vi "Gaussian Filter(Pic1 Level1).vi"(1 "Memory In":refnum<k21>, 2 "Data In":u8, 3 "DV In":bool, 6 "Height":u16, 8 "Width":u16, 10 "Rows":u16, 12 "Cols":u16) -> (16 "DV out":bool, 17 "Data Out":fxp<+,8,8>)   [LabVIEW 2016]
uses:
  <vilib>/rvi/DataTransferAndStorage/Container/Common/niFpgaContainerExecOnDevCompGetState.vi
  <vilib>/rvi/Emulation/niFpgaEmulationIsFPGAContextNoSignature.vi
  <vilib>/rvi/DataTransferAndStorage/Container/Common/niFpgaContainerGetUniqueNameForEmu.vi
  <vilib>/rvi/Emulation/niFpgaProcessEmulError.vi
  <vilib>/rvi/Emulation/niFpgaSctlEmulationGetInTimedLoop.vi
  <vilib>/rvi/errors/nirviReportUnexpectedCaseInternalError (U32).vi
  <vilib>/rvi/Memory/Memory_Emulation/niFpgaMemoryEmulationCacheClearOnFirstRun.vi
  <vilib>/rvi/Memory/Memory_Emulation/nirvimemoryEmulationManagerCache_MakeExclusive.vi
  <vilib>/rvi/Memory/Memory_Emulation/niFpgaMemoryEmulationValidateCache.vi
  <vilib>/rvi/Memory/Memory_Emulation/nirvimemoryEmulationManagerCache_InsertValue.vi
  <vilib>/Utility/error.llb/Clear Errors.vi
  <vilib>/rvi/Memory/Memory_Emulation/nirvimemoryEmulationManagerCache_ReleaseExclusive.vi
  <vilib>/rvi/Memory/Memory_Emulation/nirvimemoryEmulationManagerCache_GetValue.vi
  <vilib>/rvi/Memory/Memory_Emulation/nirvimemoryEmulationManagerCache_SetValue.vi
  <vilib>/rvi/Emulation/niFpgaSctlEmulationResourceMgr.vi
  <vilib>/rvi/DataTransferAndStorage/Container/XNode/niFpgaContainer.xnode
  <vilib>/rvi/Memory/Memory_Emulation/niFpgaMemoryEmulationRefIn.vi
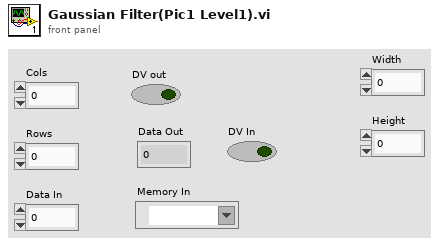
[diagram p1: front panel]
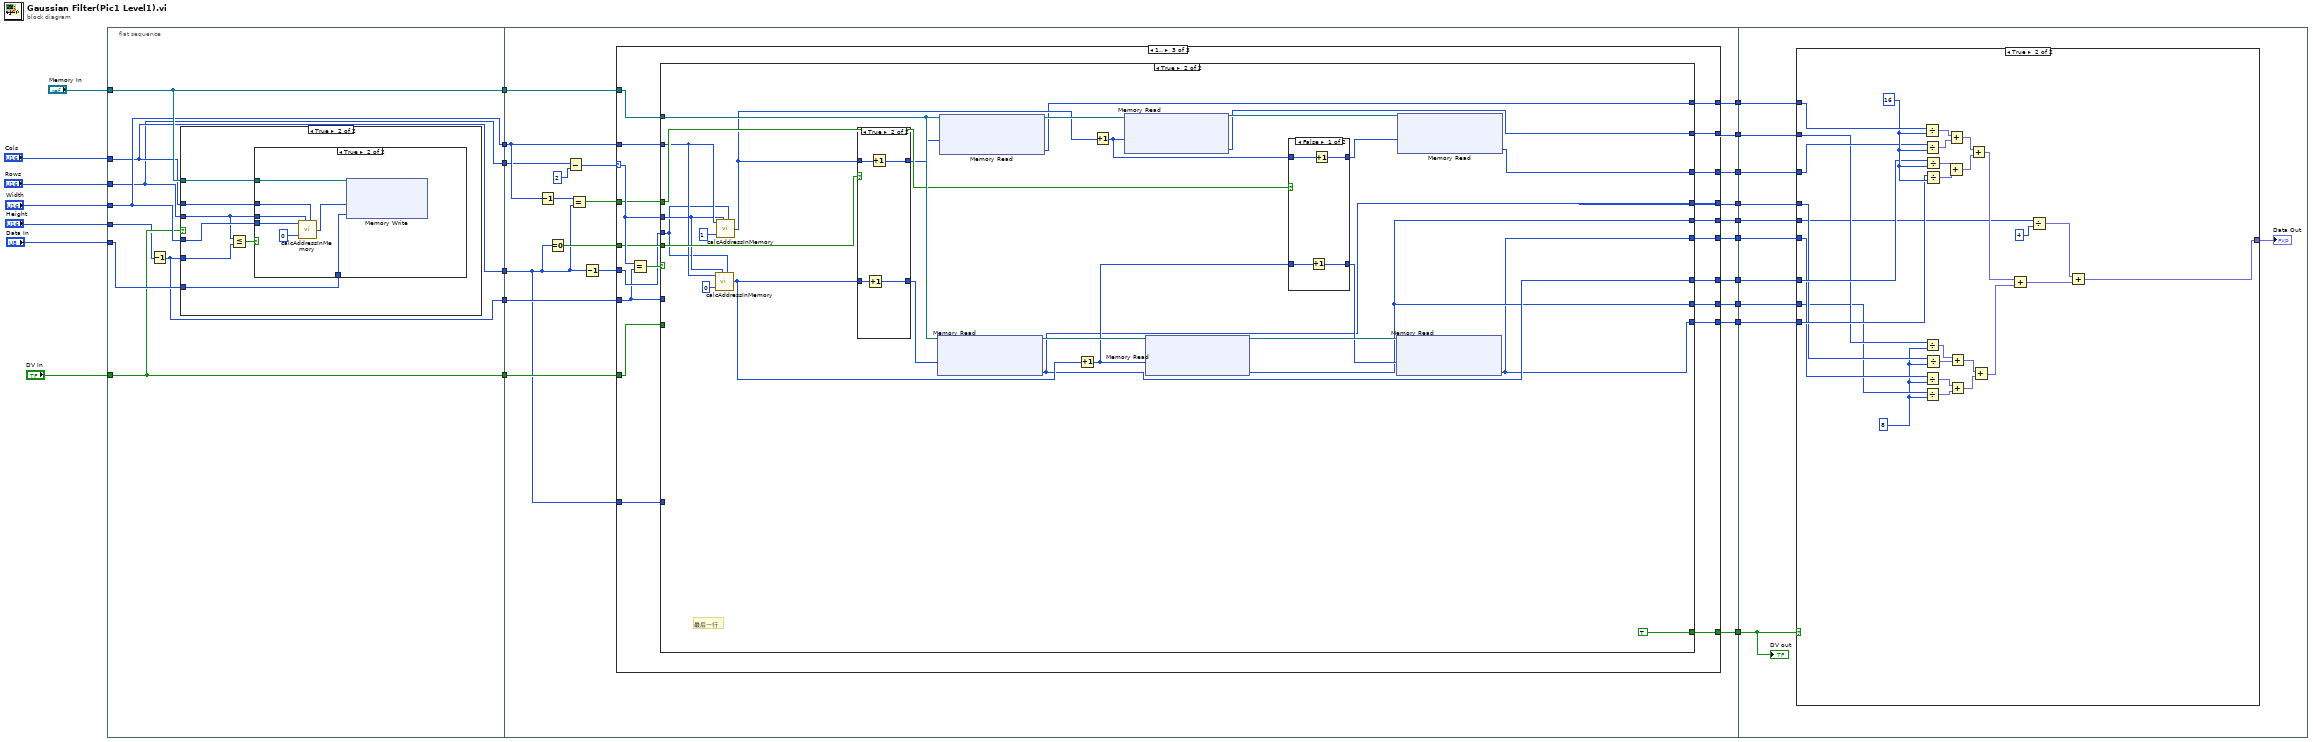
[diagram p0: block diagram]
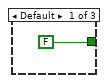
[diagram p4: hidden frame]
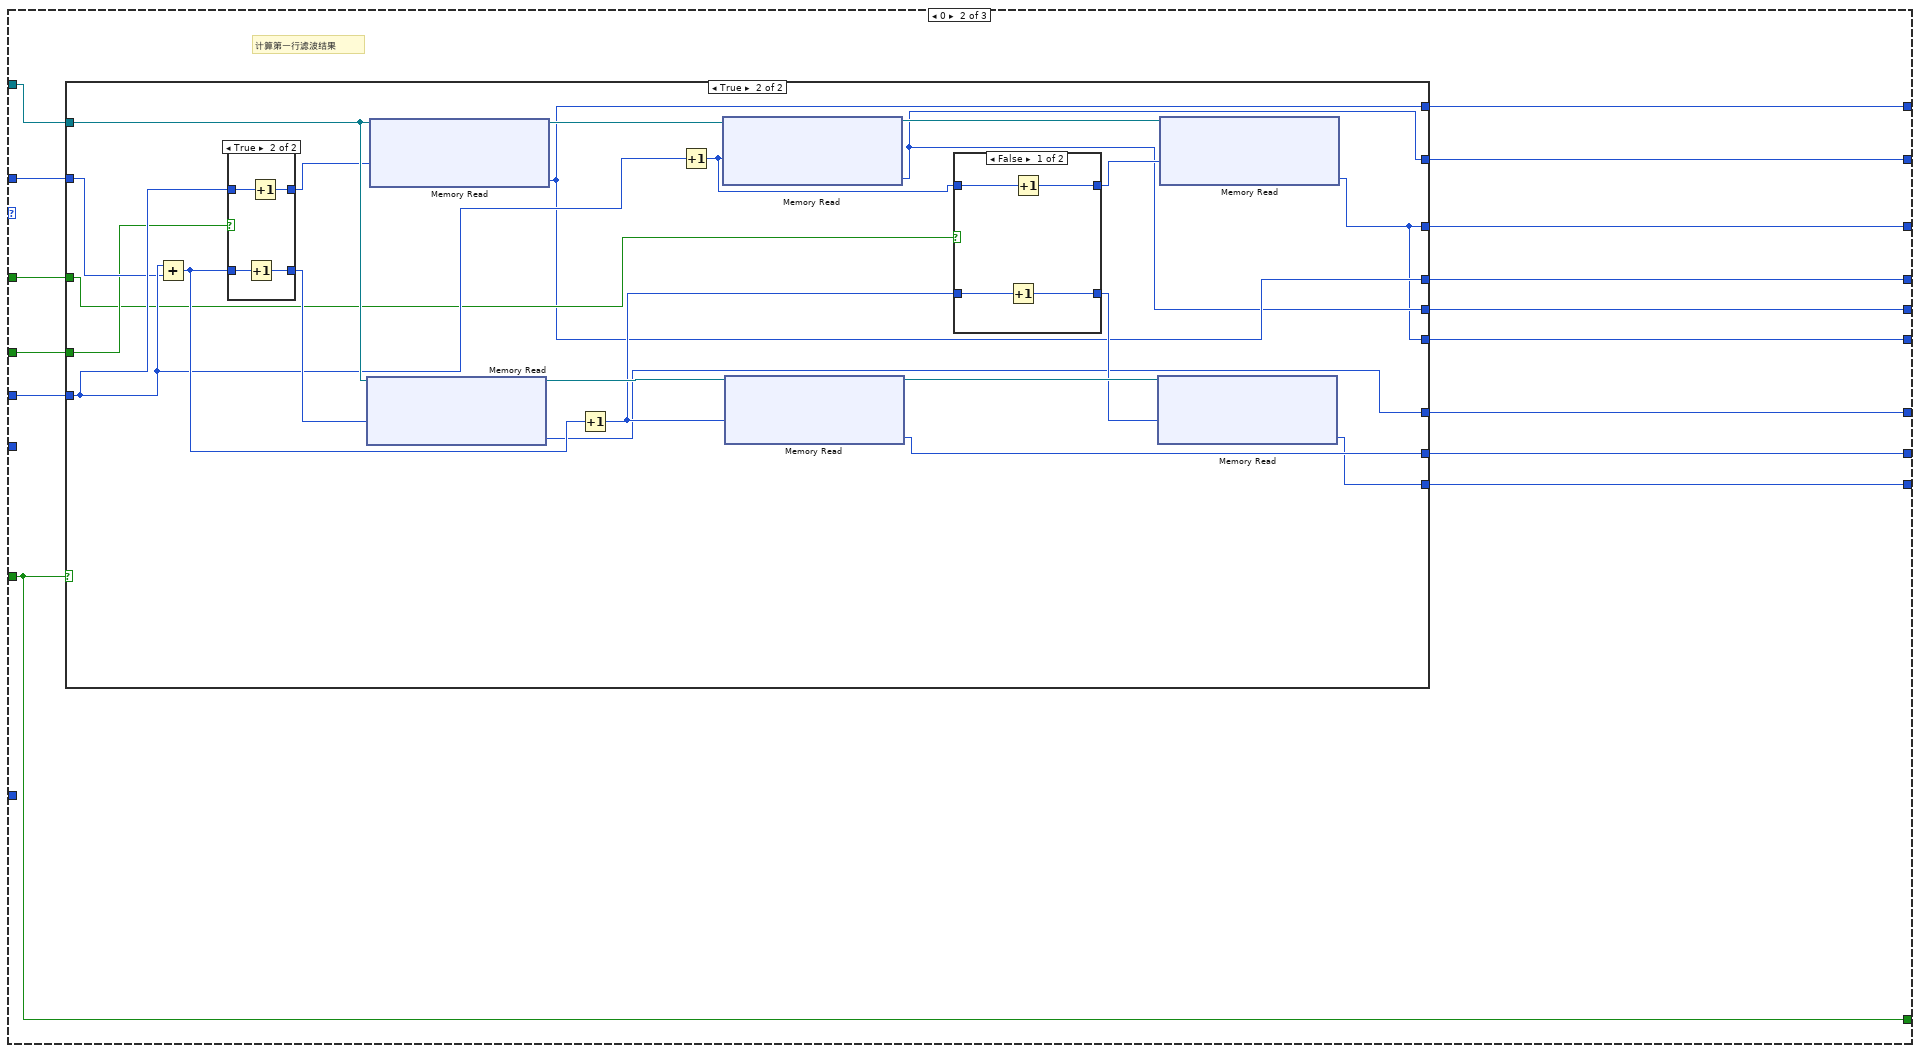
[diagram p5: hidden frame]
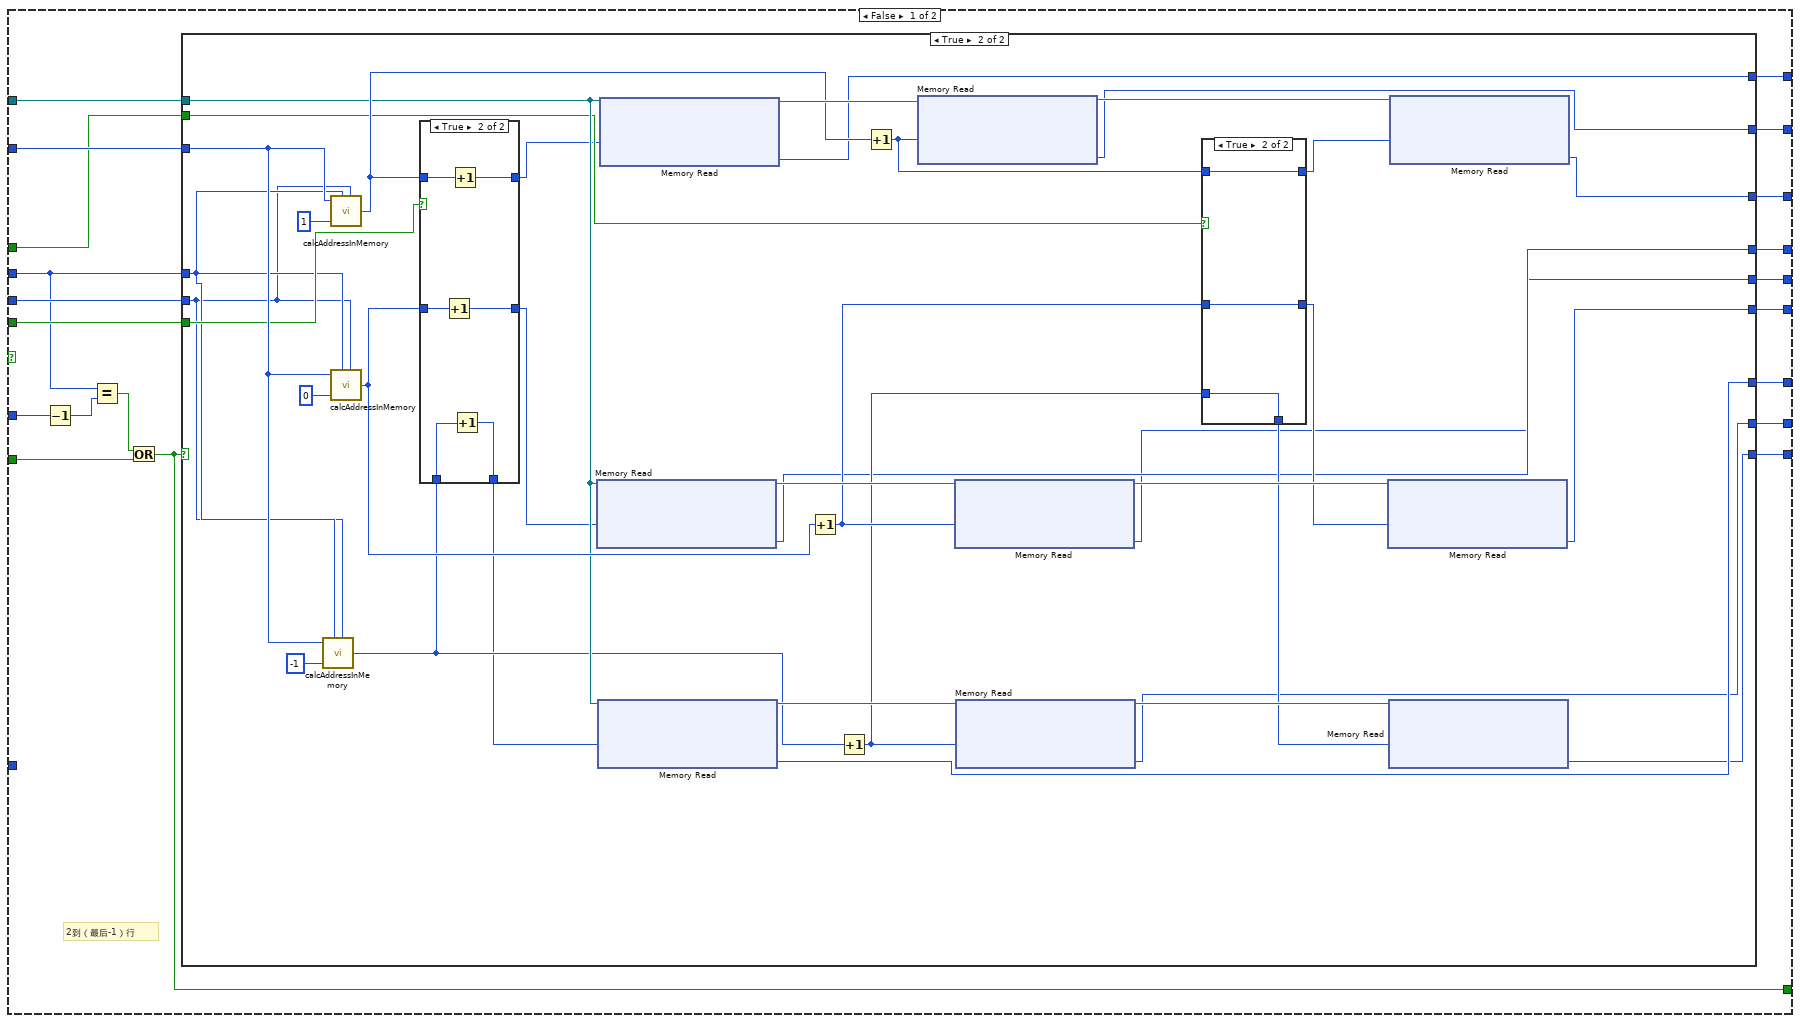
[diagram p9: hidden frame]
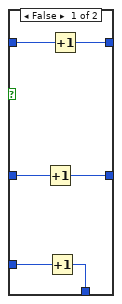
[diagram p11: hidden frame]
diagram:
  n1 = flat-sequence {
    tunnel: [w27] -> w23
    tunnel: [w29] -> w22
    tunnel: [w28] -> w21
    tunnel: [w30] -> w20
    tunnel: [w24] -> w19
    tunnel: [w26] -> w18
    tunnel: "Rows" -> [w27]
    tunnel: "Memory In" -> [w30]
    tunnel: "Cols" -> [w28]
    tunnel: "Data In" -> [w31]
    tunnel: "Width" -> [w29]
    tunnel: "Height" -> [w25]
    tunnel: "DV In" -> [w26]
    tunnel: w23 -> [w49]
    tunnel: w22 -> [w63]
    tunnel: w21 -> [w46]
    tunnel: w20 -> [w67]
    tunnel: w19 -> [w47]
    tunnel: w18 -> [w66]
    tunnel: [w61] -> w10
    tunnel: [w60] -> w9
    tunnel: [w59] -> w8
    tunnel: [w58] -> w7
    tunnel: [w57] -> w6
    tunnel: [w56] -> w5
    tunnel: [w55] -> w4
    tunnel: [w54] -> w3
    tunnel: [w53] -> w2
    tunnel: [w52] -> w1
    tunnel: w10 -> [w260]
    tunnel: w9 -> [w259]
    tunnel: w8 -> [w255]
    tunnel: w7 -> [w258]
    tunnel: w6 -> [w254]
    tunnel: w5 -> [w253]
    tunnel: w4 -> [w252]
    tunnel: w3 -> [w257]
    tunnel: w2 -> [w251]
    tunnel: w1 -> [w256]
    frame #0 {
      n2 = Decrement(x=w25) -> (x-1=w24:u16)
      n3 = case shown="True" w26 {
        tunnel: w31 -> [_ w38]
        tunnel: w27 -> [_ w32]
        tunnel: w29 -> [_ w37]
        tunnel: w28 -> [_ w36]
        tunnel: w30 -> [_ w35]
        tunnel: w24 -> [_ w33]
        frame False {
        }
        frame True {
          n4 = Less Or Equal?(x=w32, y=w33) -> (x <= y?=w34:bool)
          n5 = case shown="True" w34 {
            tunnel: w38 -> [_ w45]
            tunnel: w32 -> [_ w44]
            tunnel: w37 -> [_ w43]
            tunnel: w36 -> [_ w42]
            tunnel: w35 -> [_ w41]
            frame False {
            }
            frame True {
              n6 = call "calcAddressInMemory.vi"("Width"=w43, "Rows"=w44, "delayRowCount"=i16 0, "Cols"=w42) -> ("addressInMemory"=w40:u16)  [unwired: 5 in]
              n7 = xnode ("Memory Write")("Address"=w40, "Data"=w45, "Memory In"=w41) -> ()  [unwired: 1 out]
            }
          }
        }
      }
    }
    frame #1 {
      n8 = Decrement(x=w63) -> (x-1=w62:u16)
      n9 = Equal To 0?(x=w46) -> (x = 0?=w65:bool)
      n10 = Subtract(x=w49, y=i16 2 ("delayRowCount")) -> (x-y=w51:u16)
      n11 = Equal?(x=w62, y=w46) -> (x = y?=w64:bool)
      n12 = Decrement(x=w46) -> (x-1=w50:u16)
      n13 = case shown="1.." w51 {
        selector: w51 -> [_ _ w136]
        tunnel: w67 -> [_ w83 w135]
        tunnel: w50 -> [_ w82 w131]
        tunnel: w63 -> [_ w81 w132]
        tunnel: w47 -> [_ _ w119]
        tunnel: w66 -> [_ w78 w120]
        tunnel: w65 -> [_ w80 w133]
        tunnel: w64 -> [_ w79 w134]
        tunnel: [FALSE w78 w121] -> w61
        tunnel: [_ w77 w130] -> w60
        tunnel: [_ w76 w129] -> w59
        tunnel: [_ w75 w128] -> w58
        tunnel: [_ w74 w127] -> w57
        tunnel: [_ w73 w126] -> w56
        tunnel: [_ w72 w125] -> w55
        tunnel: [_ w71 w124] -> w54
        tunnel: [_ w70 w123] -> w53
        tunnel: [_ w69 w122] -> w52
        tunnel: w46 -> [_ _ w118]
        frame Default {
        }
        frame 0 {
          # "计算第一行滤波结果"
          n14 = case shown="True" w78 {
            tunnel: w83 -> [_ w102]
            tunnel: w82 -> [_ w93]
            tunnel: w81 -> [_ w92]
            tunnel: w80 -> [_ w91]
            tunnel: w79 -> [_ w90]
            tunnel: [_ w89] -> w77
            tunnel: [_ w88] -> w76
            tunnel: [_ w87] -> w75
            tunnel: [_ w89] -> w74
            tunnel: [_ w88] -> w73
            tunnel: [_ w87] -> w72
            tunnel: [_ w86] -> w71
            tunnel: [_ w85] -> w70
            tunnel: [_ w84] -> w69
            frame False {
            }
            frame True {
              n15 = Add(x=w93, y=w92) -> (x+y=w95:u16)
              n16 = case shown="True" w91 {
                tunnel: w93 -> [w113 w117]
                tunnel: [w113 w116] -> w96
                tunnel: w95 -> [w112 w115]
                tunnel: [w112 w114] -> w94
                frame False {
                }
                frame True {
                  n17 = Increment(x=w115) -> (x+1=w114:u16)
                  n18 = Increment(x=w117) -> (x+1=w116:u16)
                }
              }
              n19 = xnode "Memory Read"("Address"=w94, "Memory In"=w102) -> ("Data"=w86:u8, "Memory Out"=w101:refnum<k21>)
              n20 = xnode "Memory Read"("Address"=w96, "Memory In"=w102) -> ("Data"=w89:u8, "Memory Out"=w105:refnum<k21>)
              n21 = Increment(x=w95) -> (x+1=w97:u16)
              n22 = Increment(x=w93) -> (x+1=w98:u16)
              n23 = xnode "Memory Read"("Address"=w98, "Memory In"=w105) -> ("Data"=w88:u8, "Memory Out"=w104:refnum<k21>)
              n24 = xnode "Memory Read"("Address"=w97, "Memory In"=w101) -> ("Data"=w85:u8, "Memory Out"=w100:refnum<k21>)
              n25 = case shown="False" w90 {
                tunnel: [w109 w111] -> w103
                tunnel: [w108 w110] -> w99
                tunnel: w98 -> [w107 w111]
                tunnel: w97 -> [w106 w110]
                frame False {
                  n26 = Increment(x=w106) -> (x+1=w108:u16)
                  n27 = Increment(x=w107) -> (x+1=w109:u16)
                }
                frame True {
                }
              }
              n28 = xnode "Memory Read"("Address"=w99, "Memory In"=w100) -> ("Data"=w84:u8)  [unwired: 1 out]
              n29 = xnode "Memory Read"("Address"=w103, "Memory In"=w104) -> ("Data"=w87:u8)  [unwired: 1 out]
            }
          }
        }
        frame 1.. {
          n30 = Equal?(x=w136, y=w119) -> (x = y?=w137:bool)
          n31 = case shown="True" w137 {
            tunnel: w136 -> [w140 w228]
            tunnel: w135 -> [w157 w234]
            tunnel: w134 -> [w144 w233]
            tunnel: w133 -> [w145 w232]
            tunnel: w132 -> [w155 w229]
            tunnel: w131 -> [w156 w227]
            tunnel: [w154 w217] -> w130
            tunnel: [w153 w216] -> w129
            tunnel: [w152 w215] -> w128
            tunnel: [w151 w214] -> w127
            tunnel: [w150 w213] -> w126
            tunnel: [w149 w212] -> w125
            tunnel: [w148 w214] -> w124
            tunnel: [w147 w213] -> w123
            tunnel: [w146 w212] -> w122
            tunnel: [w143 TRUE] -> w121
            tunnel: w120 -> [w142 _]
            tunnel: w119 -> [w138 _]
            tunnel: w118 -> [_ _]
            frame False {
              # "2到（最后-1）行"
              n32 = Decrement(x=w138) -> (x-1=w139:u16)
              n33 = Equal?(x=w140, y=w139) -> (x = y?=w141:bool)
              n34 = Or(x=w141, y=w142) -> (x .or. y?=w143:bool)
              n35 = case shown="True" w143 {
                tunnel: w157 -> [_ w182]
                tunnel: w156 -> [_ w158]
                tunnel: w155 -> [_ w180]
                tunnel: w140 -> [_ w159]
                tunnel: [_ w168] -> w154
                tunnel: [_ w167] -> w153
                tunnel: [_ w166] -> w152
                tunnel: [_ w165] -> w151
                tunnel: [_ w164] -> w150
                tunnel: [_ w163] -> w149
                tunnel: [_ w162] -> w148
                tunnel: [_ w161] -> w147
                tunnel: [_ w160] -> w146
                tunnel: w145 -> [_ w179]
                tunnel: w144 -> [_ w178]
                frame False {
                }
                frame True {
                  n36 = call "calcAddressInMemory.vi"("Width"=w180, "Rows"=w159, "delayRowCount"=i16 -1, "Cols"=w158) -> ("addressInMemory"=w181:u16)  [unwired: 5 in]
                  n37 = call "calcAddressInMemory.vi"("Width"=w180, "Rows"=w159, "delayRowCount"=i16 1, "Cols"=w158) -> ("addressInMemory"=w186:u16)  [unwired: 5 in]
                  n38 = call "calcAddressInMemory.vi"("Width"=w180, "Rows"=w159, "delayRowCount"=i16 0, "Cols"=w158) -> ("addressInMemory"=w187:u16)  [unwired: 5 in]
                  n39 = case shown="True" w179 {
                    tunnel: w186 -> [w205 w211]
                    tunnel: [w205 w210] -> w177
                    tunnel: w187 -> [w204 w209]
                    tunnel: [w204 w208] -> w174
                    tunnel: [w203 w207] -> w171
                    tunnel: w181 -> [w203 w206]
                    frame False {
                    }
                    frame True {
                      n40 = Increment(x=w209) -> (x+1=w208:u16)
                      n41 = Increment(x=w211) -> (x+1=w210:u16)
                      n42 = Increment(x=w206) -> (x+1=w207:u16)
                    }
                  }
                  n43 = xnode "Memory Read"("Address"=w174, "Memory In"=w182) -> ("Data"=w165:u8, "Memory Out"=w191:refnum<k21>)
                  n44 = xnode "Memory Read"("Address"=w171, "Memory In"=w182) -> ("Data"=w162:u8, "Memory Out"=w184:refnum<k21>)
                  n45 = xnode "Memory Read"("Address"=w177, "Memory In"=w182) -> ("Data"=w168:u8, "Memory Out"=w193:refnum<k21>)
                  n46 = Increment(x=w187) -> (x+1=w173:u16)
                  n47 = Increment(x=w181) -> (x+1=w170:u16)
                  n48 = Increment(x=w186) -> (x+1=w176:u16)
                  n49 = xnode "Memory Read"("Address"=w176, "Memory In"=w193) -> ("Data"=w167:u8, "Memory Out"=w192:refnum<k21>)
                  n50 = xnode "Memory Read"("Address"=w173, "Memory In"=w191) -> ("Data"=w164:u8, "Memory Out"=w190:refnum<k21>)
                  n51 = xnode "Memory Read"("Address"=w170, "Memory In"=w184) -> ("Data"=w161:u8, "Memory Out"=w183:refnum<k21>)
                  n52 = case shown="True" w178 {
                    tunnel: [w199 w202] -> w175
                    tunnel: [w198 w201] -> w172
                    tunnel: w176 -> [w197 w202]
                    tunnel: w173 -> [w196 w201]
                    tunnel: w170 -> [w195 w200]
                    tunnel: [w194 w200] -> w169
                    frame False {
                      n53 = Increment(x=w196) -> (x+1=w198:u16)
                      n54 = Increment(x=w195) -> (x+1=w194:u16)
                      n55 = Increment(x=w197) -> (x+1=w199:u16)
                    }
                    frame True {
                    }
                  }
                  n56 = xnode "Memory Read"("Address"=w172, "Memory In"=w190) -> ("Data"=w163:u8)  [unwired: 1 out]
                  n57 = xnode "Memory Read"("Address"=w169, "Memory In"=w183) -> ("Data"=w160:u8)  [unwired: 1 out]
                  n58 = xnode "Memory Read"("Address"=w175, "Memory In"=w192) -> ("Data"=w166:u8)  [unwired: 1 out]
                }
              }
            }
            frame True {
              # "最后一行"
              n59 = call "calcAddressInMemory.vi"("Width"=w229, "Rows"=w228, "delayRowCount"=i16 0, "Cols"=w227) -> ("addressInMemory"=w226:u16)  [unwired: 5 in]
              n60 = call "calcAddressInMemory.vi"("Width"=w229, "Rows"=w228, "delayRowCount"=i16 1, "Cols"=w227) -> ("addressInMemory"=w225:u16)  [unwired: 5 in]
              n61 = case shown="True" w232 {
                tunnel: w225 -> [w246 w250]
                tunnel: [w246 w249] -> w223
                tunnel: w226 -> [w245 w248]
                tunnel: [w245 w247] -> w220
                frame False {
                }
                frame True {
                  n62 = Increment(x=w248) -> (x+1=w247:u16)
                  n63 = Increment(x=w250) -> (x+1=w249:u16)
                }
              }
              n64 = xnode "Memory Read"("Address"=w220, "Memory In"=w234) -> ("Data"=w214:u8, "Memory Out"=w236:refnum<k21>)
              n65 = xnode "Memory Read"("Address"=w223, "Memory In"=w234) -> ("Data"=w217:u8, "Memory Out"=w238:refnum<k21>)
              n66 = Increment(x=w226) -> (x+1=w219:u16)
              n67 = Increment(x=w225) -> (x+1=w222:u16)
              n68 = xnode "Memory Read"("Address"=w222, "Memory In"=w238) -> ("Data"=w216:u8, "Memory Out"=w237:refnum<k21>)
              n69 = xnode "Memory Read"("Address"=w219, "Memory In"=w236) -> ("Data"=w213:u8, "Memory Out"=w235:refnum<k21>)
              n70 = case shown="False" w233 {
                tunnel: [w242 w244] -> w221
                tunnel: [w241 w243] -> w218
                tunnel: w222 -> [w240 w244]
                tunnel: w219 -> [w239 w243]
                frame False {
                  n71 = Increment(x=w239) -> (x+1=w241:u16)
                  n72 = Increment(x=w240) -> (x+1=w242:u16)
                }
                frame True {
                }
              }
              n73 = xnode "Memory Read"("Address"=w218, "Memory In"=w235) -> ("Data"=w212:u8)  [unwired: 1 out]
              n74 = xnode "Memory Read"("Address"=w221, "Memory In"=w237) -> ("Data"=w215:u8)  [unwired: 1 out]
            }
          }
        }
      }
    }
    frame #2 {
      n75 = case shown="True" w260 {
        tunnel: [_ w262] -> w261
        tunnel: w259 -> [_ w273]
        tunnel: w258 -> [_ w271]
        tunnel: w257 -> [_ w270]
        tunnel: w256 -> [_ w269]
        tunnel: w255 -> [_ w268]
        tunnel: w254 -> [_ w267]
        tunnel: w253 -> [_ w263]
        tunnel: w252 -> [_ w266]
        tunnel: w251 -> [_ w265]
        frame False {
        }
        frame True {
          w264 = u8 8 ("y")
          w272 = u8 16 ("y")
          n76 = Divide(x=w273, y=w272) -> (x/y=w290:fxp<+,4,4>)
          n77 = Divide(x=w271, y=w272) -> (x/y=w289:fxp<+,4,4>)
          n78 = Divide(x=w268, y=w264) -> (x/y=w284:fxp<+,5,5>)
          n79 = Divide(x=w266, y=w264) -> (x/y=w286:fxp<+,5,5>)
          n80 = Divide(x=w265, y=w264) -> (x/y=w285:fxp<+,5,5>)
          n81 = Divide(x=w270, y=w272) -> (x/y=w288:fxp<+,4,4>)
          n82 = Divide(x=w269, y=w272) -> (x/y=w287:fxp<+,4,4>)
          n83 = Divide(x=w267, y=w264) -> (x/y=w283:fxp<+,5,5>)
          n84 = Add(x=w288, y=w287) -> (x+y=w276:fxp<+,5,5>)
          n85 = Add(x=w290, y=w289) -> (x+y=w277:fxp<+,5,5>)
          n86 = Add(x=w284, y=w283) -> (x+y=w275:fxp<+,6,6>)
          n87 = Add(x=w286, y=w285) -> (x+y=w274:fxp<+,6,6>)
          n88 = Add(x=w277, y=w276) -> (x+y=w281:fxp<+,6,6>)
          n89 = Add(x=w275, y=w274) -> (x+y=w280:fxp<+,7,7>)
          n90 = Add(x=w281, y=w280) -> (x+y=w278:fxp<+,8,8>)
          n91 = Divide(x=w263, y=u8 4) -> (x/y=w279:fxp<+,6,6>)
          n92 = Add(x=w279, y=w278) -> (x+y=w262:fxp<+,8,8>)
        }
      }
      "Data Out" <- w261
      "DV out" <- w260
    }
  }
